vi "Unsubscribe.vi"(8 "error in (no error)":errorcluster, 10 "SubscriptionPolicy":T1, 11 "Mediator In":refnum<class "Mediator.lvclass">) -> (0 "error out":errorcluster, 3 "Mediator Out":refnum<class "Mediator.lvclass">)   [LabVIEW 2017, in "Mediator.lvlib" / "Mediator.lvclass"]
doc: "<License>\nCopyright © 2017 Composed Systems, LLC | All rights reserved\nwww.composed.io\n\nAuthor: Ethan Stern <ethan.stern@composed.io>\n\nThis software is provided \"AS IS\" WITHOUT WARRANTIES, either express or implied, AND IS FOR EDUCATIONAL PURPOSES ONLY.\n</License>"
uses:
  Mediator.lvclass
  IMediator/ISubscriptionPolicy/ISubscriptionPolicy Reference.ctl
  IMediator/ISubscriptionPolicy/ISubscriptionPolicy.lvclass
  Mediator.lvclass/Mediator.ctl
  Topic Messages/Remove Topic Subscriber Msg/Remove Topic Subscriber Msg.lvclass/Remove Topic Subscriber Msg.ctl
  <vilib>/ActorFramework/Message Enqueuer/Message Enqueuer.lvclass/Message Enqueuer.ctl
  <vilib>/ActorFramework/Message Enqueuer/Enqueue.vi
  Topic Messages/Remove Topic Subscriber Msg/Remove Topic Subscriber Msg.lvclass
  C:/Program Files (x86)/National Instruments/LabVIEW 2017/vi.lib/ActorFramework/Message/Message.lvclass
  <vilib>/ActorFramework/Message Priority Queue/Priority Enqueue.vi
  TopicLookupTable/TopicLookupTable.lvclass
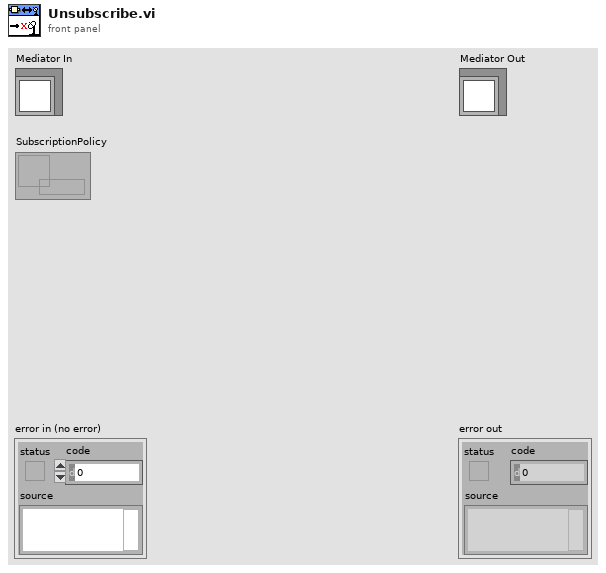
[diagram p1: front panel]
types:
  T1 = typedef "IMediator.lvlib/ISubscriptionPolicy.lvclass/ISubscriptionPolicy Reference.ctl" = refnum<data-value>
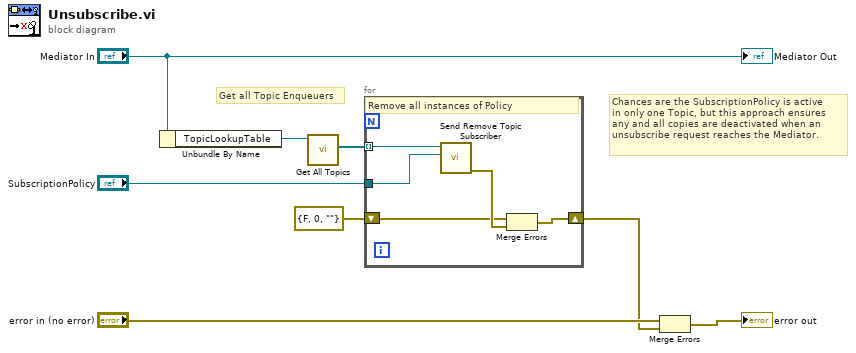
[diagram p0: block diagram]
diagram:
  # "Get all Topic Enqueuers"
  # "Chances are the SubscriptionPolicy is active\nin only one Topic, but this approach ensures\nany and all copies are deactivated when an\nunsubscribe request reaches the Mediator."
  n1 = Unbundle By Name("Mediator In") -> ("TopicLookupTable"=w6:refnum<data-value>)
  n2 = call "Get All Topics.vi"("TopicLookupTable"=w6) -> ("Topic Enqueuers"=w5:refnum<class "Message Enqueuer.lvclass">[])  [unwired: 8 in, 2 out]
  n3 = for {
    tunnel: w5 -> [w13] mode=indexing
    tunnel: "SubscriptionPolicy" -> [w12]
    shift-right: [w10] -> w1
    shift-left: errorcluster {"status"=FALSE, "code"=0, "source"=""} ("error out") -> [w9]
    # "Remove all instances of Policy"
    n4 = call "Send Remove Topic Subscriber.vi"("Subscription Policy"=w12, "Message Enqueuer"=w13) -> ("error out"=w11:errorcluster)  [unwired: 8 in, 1 out]
    n5 = Merge Errors(w9, w11) -> (w10:errorcluster)
  }
  n6 = Merge Errors("error in (no error)", w1) -> (→"error out":errorcluster)
  "Mediator Out" <- "Mediator In"
